vi "test from file.vi"() -> ()   [LabVIEW 2018, in "Data Parser.lvclass"]
uses:
  Data Parser.lvclass
panel:
  out "same":bool
  out "frame string":string
  out "<f> string":string
  out "frame num":i32
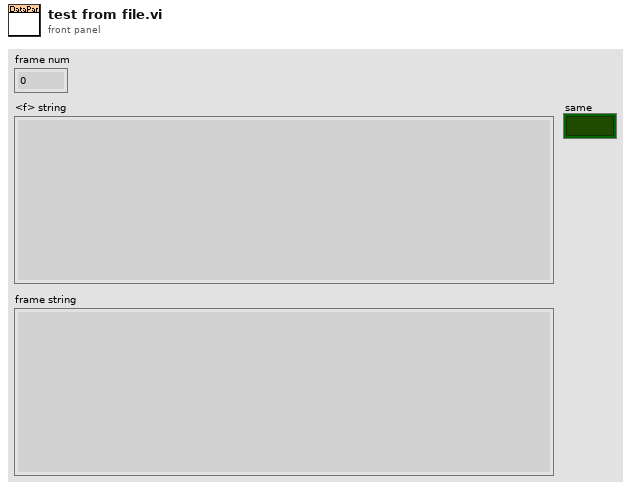
[diagram p1: front panel]
types:
  T1 = typedef "Data Parser.lvclass/frame data.ctl" = cluster{"Title":T2, "Basic Data":T3, "Sound":string, "<o> Data":T4, "<bp> Data":T5, "<c> Data":T6, "<w> Data":T7, "<i> Data Array":T8[], "<b> Data Array":T9[]}
  T2 = typedef "Data Parser.lvclass/frame title.ctl" = cluster{"number":string, "name":string}
  T3 = typedef "Data Parser.lvclass/frame basic data.ctl" = cluster{"Basic":cluster{"pic":string, "state":string, "wait":string, "next":string}, "Move":cluster{"dvx":string, "dvy":string, "dvz":string}, "Pic Center":cluster{"centerx":string, "centery":string}, "Skill":cluster{"hit_a":string, "hit_d":string, "hit_j":string, "hit_Fa":string, "hit_Ua":string, "hit_Da":string, "hit_Fj":string, "hit_Uj":string, "hit_Dj":string, "hit_ja":string}, "Mp":string}
  T4 = typedef "Data Parser.lvclass/frame o data.ctl" = cluster{"kind":string, "x":string, "y":string, "action":string, "dvx":string, "dvy":string, "dvz":string, "oid":string, "facing":string}
  T5 = typedef "Data Parser.lvclass/frame bp data.ctl" = cluster{"x":string, "y":string}
  T6 = typedef "Data Parser.lvclass/frame c data.ctl" = cluster{"kind":string, "x":string, "y":string, "injury":string, "cover":string, "vaction":string, "aaction":string, "taction":string, "hurtable":string, "decrease":string, "fronthurtact":string, "backhurtact":string, "dircontrol":string, "throwvx":string, "throwvy":string, "throwvz":string, "throwinjury":string}
  T7 = typedef "Data Parser.lvclass/frame w data.ctl" = cluster{"kind":string, "x":string, "y":string, "weaponact":string, "dvx":string, "dvy":string, "dvz":string, "attacking":string, "cover":string}
  T8 = typedef "Data Parser.lvclass/frame i data.ctl" = cluster{"kind":string, "x":string, "y":string, "w":string, "h":string, "dvx":string, "dvy":string, "dvz":string, "fall":string, "arest":string, "vrest":string, "bdefend":string, "injury":string, "zwidth":string, "effect":string, "catchingact":string, "caughtact":string}
  T9 = typedef "Data Parser.lvclass/frame b data.ctl" = cluster{"kind":string, "x":string, "y":string, "w":string, "h":string}
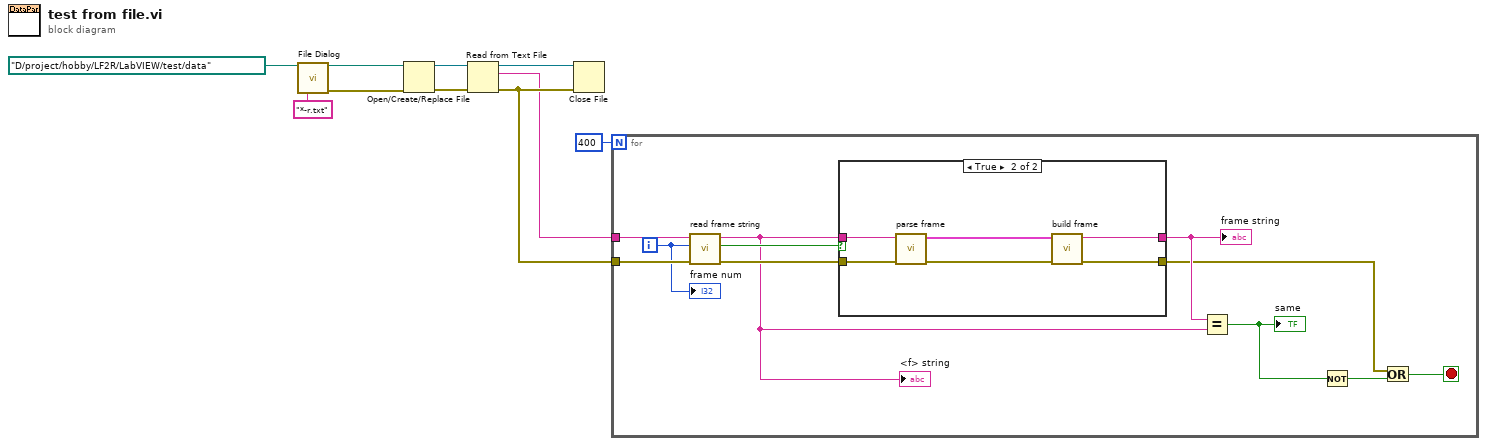
[diagram p0: block diagram]
diagram:
  n1 = call "File Dialog"("start path"=path "D:/project/hobby/LF2R/LabVIEW/test/data", "pattern (all files)"="*-r.txt") -> ("selected path"=w5:path, "error out"=w4:errorcluster)  [unwired: 10 in, 2 out]
  n2 = Open/Create/Replace File(file path (use dialog)=w5, error in=w4) -> (refnum out=w10:refnum<file>, error out=w9:errorcluster)  [unwired: 4 in, 1 out]
  n3 = Read from Text File(file (use dialog)=w10, error in=w9) -> (refnum out=w8:refnum<file>, text=w2:string, error out=w3:errorcluster)  [unwired: 2 in, 1 out]
  n4 = Close File(refnum=w8, error in=w3) -> ()  [unwired: 2 out]
  n5 = for {
    N: 400 -> [_]
    tunnel: w3 -> [w20]
    tunnel: w2 -> [w19]
    i -> [w17]
    stop <- w18 stop-if-true
    n6 = call "read frame string.vi"("error in"=w20, "frame number"=w17, "file string"=w19) -> ("error out"=w21:errorcluster, "found"=w16:bool, "<f> string"=w13:string)  [unwired: 5 in, 1 out]
    "<f> string" <- w13
    n7 = case shown="True" w16 {
      tunnel: w13 -> [w22 w27]
      tunnel: w21 -> [w23 w26]
      tunnel: [w22 w25] -> w15
      tunnel: [w23 w24] -> w14
      frame False {
      }
      frame True {
        n8 = call "parse frame.vi"("error in (no error)"=w26, "<f> string"=w27) -> ("error out"=w28:errorcluster, "frame data"=w29:T1)  [unwired: 8 in]
        n9 = call "build frame.vi"("error in (no error)"=w28, "frame data"=w29) -> ("error out"=w24:errorcluster, "<f> string"=w25:string)  [unwired: 8 in]
      }
    }
    "frame string" <- w15
    n10 = Equal?(x=w15, y=w13) -> (x = y?=w12:bool)
    "same" <- w12
    n11 = Not(x=w12) -> (.not. x?=w11:bool)
    n12 = Or(x=w14, y=w11) -> (x .or. y?=w18:bool)
    "frame num" <- w17
  }
